vi "DelayGeneratorTrack.vi"(8 "error in (no error)":errorcluster) -> (0 "error out":errorcluster)   [LabVIEW 2009]
uses:
  Controls/DelayGeneratorCommand.ctl
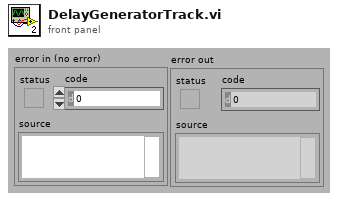
[diagram p1: front panel]
types:
  T1 = typedef "DelayGeneratorCommand.ctl" = enum16{"IDLE", "TRACK", "QUIT"}
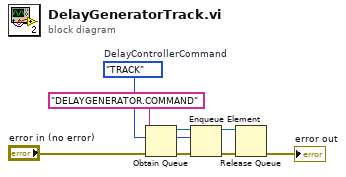
[diagram p0: block diagram]
diagram:
  w4 = DelayGeneratorCommand."TRACK"  # DelayControllerCommand
  n1 = Obtain Queue(name (unnamed)="DELAYGENERATOR.COMMAND", element data type=w4, error in (no error)="error in (no error)") -> (queue out=w5:refnum<queue>, error out=w6:errorcluster)  [unwired: 2 in, 1 out]
  n2 = Enqueue Element(queue=w5, element=w4, error in (no error)=w6) -> (queue out=w3:refnum<queue>, error out=w2:errorcluster)  [unwired: 1 in, 1 out]
  n3 = Release Queue(queue=w3, error in (no error)=w2) -> (error out=→"error out":errorcluster)  [unwired: 1 in, 2 out]
